vi "(SubVI) Initiate Queue, Image and File Opening.vi"(11 "Path String Array":string[](array[string])) -> (0 "error out":errorcluster, 1 "Refnum out":T1, 2 "Byte Stream File out":refnum<file>, 3 "Queue out":refnum<queue>, 4 "Image Buffer":T1[](array[typedef]), 5 "# Of Buffers":i32)   [LabVIEW 2014]
uses:
  <vilib>/vision/Image Controls.llb/IMAQ Image.ctl
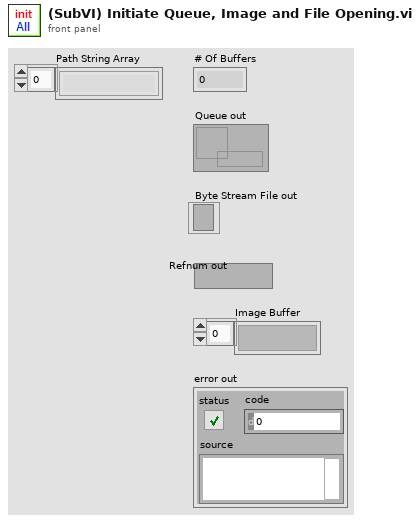
[diagram p1: front panel]
types:
  T1 = typedef "IMAQ Image.ctl" = refnum<image>
  T2 = typedef "Image Type" = u32
  T3 = cluster{"Grab Image":T1, "max queue size (-1, unlimited)":u32}
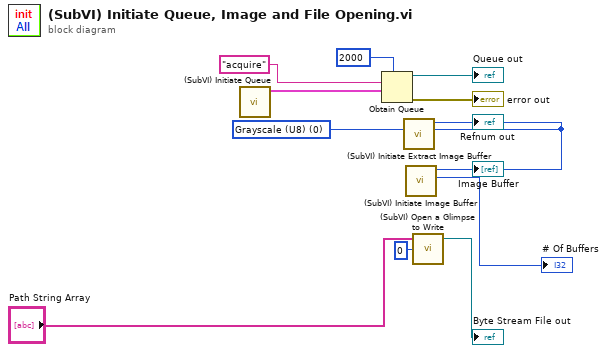
[diagram p0: block diagram]
diagram:
  w9 = T2 0 items=["Grayscale (U8)", "Grayscale (I16)", "Grayscale (SGL)", "Complex (CSG)", "RGB (U32)", "HSL (U32)", "RGB (U64)", "Grayscale (U16)"] ("Image Type")
  n1 = call "(SubVI) Initiate Queue.vi"() -> ("Cluster"=w5:T3)  [unwired: 11 in]
  n2 = Obtain Queue(max queue size (-1, unlimited)=2000, name (unnamed)="acquire", element data type=w5) -> (queue out=→"Queue out":refnum<queue>, error out=→"error out":errorcluster)  [unwired: 2 in, 1 out]
  n3 = call "(SubVI) Initiate Extract Image Buffer.vi"("Image Type"=w9) -> ("Refnum out"=→"Refnum out":T1)  [unwired: 10 in]
  n4 = call "(SubVI) Initiate Image Buffer.vi"("Image Type"=w9) -> ("# Of Buffers"=→"# Of Buffers":i32, "Image Buffer"=→"Image Buffer":T1[])  [unwired: 9 in]
  n5 = call "(SubVI) Open a Glimpse to Write.vi"("index file (0,1,2,...)"=0, "String Path Array"="Path String Array") -> ("Byte Stream File out"=→"Byte Stream File out":refnum<file>)  [unwired: 2 in, 1 out]
